vi "nominal workbook get batch.vi"(7 "out_count":u32, 8 "error in (no error)":errorcluster, 9 "out_list":i32, 10 "rid_list":i32, 11 "client":i32) -> (0 "error out":errorcluster, 1 "out_list out":i32, 3 "function return":i32, 5 "out_count out":u32)   [LabVIEW 2020, in "client.lvlib"]
doc: "int32_t nominal_workbook_get_batch(int32_t client,\n int32_t rid_list,\n int32_t *out_list,\n uint32_t *out_count);"
uses:
  client.lvlib
  bin/nominalClient_64.dll
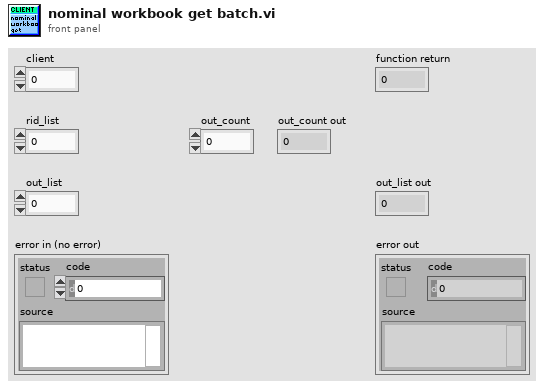
[diagram p1: front panel]
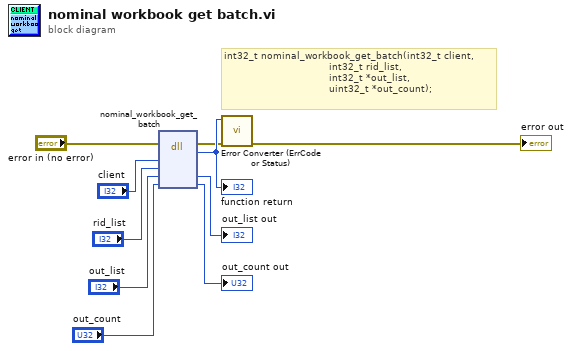
[diagram p0: block diagram]
diagram:
  # "int32_t nominal_workbook_get_batch(int32_t client,\n                                   int32_t rid_list,\n                                   int32_t *out_list,\n                                   uint32_t *out_count);"
  n1 = dll-call lib="C:/code/labview-client-rs/lv_src/bin/nominalClient_*.*" fn="nominal_workbook_get_batch"(error in="error in (no error)", "client"="client", "rid_list"="rid_list", "out_list"="out_list", "out_count"="out_count") -> (error out=w2:errorcluster, w10:i32, "out_list"=→"out_list out":i32, "out_count"=→"out_count out":u32)  [unwired: 4 in, 1 out]
  "function return" <- w10
  n2 = call "Error Converter (ErrCode or Status).vi"("error in (no error)"=w2, "error code"=w10) -> ("error out"=→"error out":errorcluster)  [unwired: 9 in]
